vi "SetupMenu.vi"(8 "error in (no error)":errorcluster, 10 "MenuItemDisablesList":T1[](array[typedef]), 11 "MenuDisableCol in":refnum<class "MenuDisableCol.lvclass">) -> (0 "error out":errorcluster, 3 "MenuDisableCol out":refnum<class "MenuDisableCol.lvclass">)   [LabVIEW 2013, in "MenuDisableCol.lvclass"]
uses:
  MenuDisableCol.lvclass
  MenuItemDisables.ctl
  MenuDisableCol.lvclass/MenuDisableCol.ctl
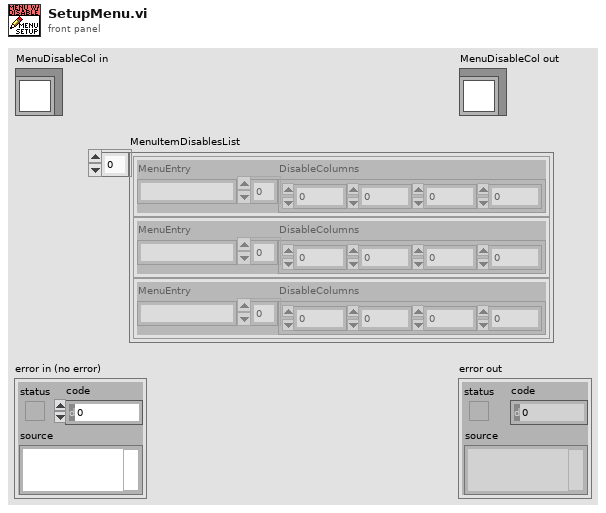
[diagram p1: front panel]
types:
  T1 = typedef "MenuItemDisables.ctl" = cluster{"MenuEntry":string, "DisableColumns":i32[]}
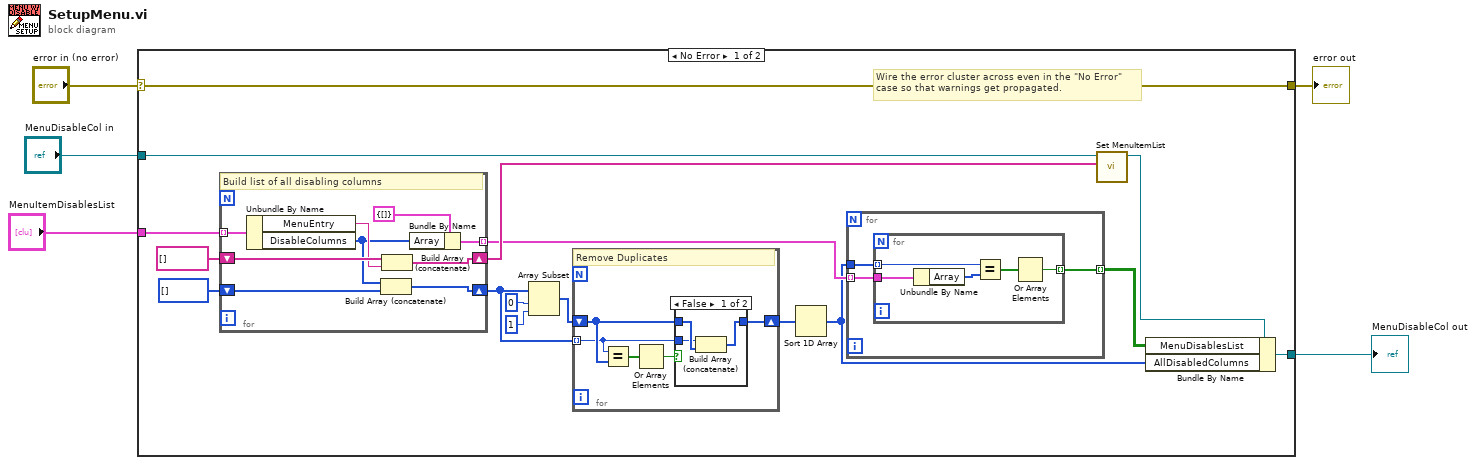
[diagram p0: block diagram]
diagram:
  n1 = case shown="No Error" "error in (no error)" {
    selector: "error in (no error)" -> [w21 w49]
    tunnel: [w21 w49] -> w4
    tunnel: [w18 w48] -> w2
    tunnel: "MenuDisableCol in" -> [w20 w48]
    tunnel: "MenuItemDisablesList" -> [w15 _]
    frame No Error {
      # "Wire the error cluster across even in the \"No Error\"\ncase so that warnings get propagated."
      n2 = for {
        shift-right: [w46] -> w16
        shift-left: string[] [] ("MenuItemList") -> [w47]
        tunnel: w15 -> [w45] mode=indexing
        tunnel: [w42] -> w8 mode=indexing
        shift-right: [w40] -> w13
        shift-left: i32[] [] -> [w39]
        # "Build list of all disabling columns"
        n3 = Unbundle By Name(w45) -> ("MenuEntry"=w44:string, "DisableColumns"=w41:i32[])
        n4 = Build Array (concatenate)(w41, w39) -> (w40:i32[])
        n5 = Build Array (concatenate)(w47, w44) -> (w46:string[])
        n6 = Bundle By Name(cluster=cluster{"Array":i32[]} {"Array"=[]} ("MenuDisables"), "Array"=w41) -> (w42:cluster{"Array":i32[]})
      }
      n7 = Array Subset(array=w13, index=0, length=1) -> (w10:i32[])
      n8 = for {
        tunnel: w13 -> [w30] mode=indexing
        shift-right: [w32] -> w9
        shift-left: w10 -> [w33]
        # "Remove Duplicates"
        n9 = Equal?(x=w30, y=w33) -> (x = y?=w34:bool[])
        n10 = Or Array Elements(Boolean array=w34) -> (logical OR=w31:bool)
        n11 = case shown="False" w31 {
          tunnel: w33 -> [w37 w38]
          tunnel: [w35 w38] -> w32
          tunnel: w30 -> [w36 _]
          frame False {
            n12 = Build Array (concatenate)(w36, w37) -> (w35:i32[])
          }
          frame True {
          }
        }
      }
      n13 = Sort 1D Array(array=w9) -> (sorted array=w7:i32[])
      n14 = for {
        tunnel: w8 -> [w23] mode=indexing
        tunnel: w7 -> [w24]
        tunnel: [w22] -> w6 mode=indexing
        n15 = for {
          tunnel: w24 -> [w29] mode=indexing
          tunnel: w23 -> [w28]
          tunnel: [w25] -> w22 mode=indexing
          n16 = Unbundle By Name(w28) -> ("Array"=w27:i32[])
          n17 = Equal?(x=w29, y=w27) -> (x = y?=w26:bool[])
          n18 = Or Array Elements(Boolean array=w26) -> (logical OR=w25:bool)
        }
      }
      n19 = call-dynamic "Set MenuItemList.vi"("MenuItemList"=w16, "MenuCol in"=w20) -> ("MenuCol out"=w19:refnum<class "MenuDisableCol.lvclass">)  [unwired: 8 in, 1 out]
      n20 = Bundle By Name(cluster=w19, "MenuDisablesList"=w6, "AllDisabledColumns"=w7) -> (w18:refnum<class "MenuDisableCol.lvclass">)
    }
    frame Error {
    }
  }
  "error out" <- w4
  "MenuDisableCol out" <- w2
